vi "标准状态机.vi"(7 "Stop":bool, 8 "error in (no error)":errorcluster caption="错误输入（无错误）", 11 "Start":bool) -> (0 "error out":errorcluster caption="错误输出", 3 "Status":T1={"State"=enum."Idle", "Motor"={"#1"=FALSE, "#2"=FALSE, "#3"=FALSE}, "Timer"=30.0})   [LabVIEW 2013]
uses:
  Control/Data.ctl
  Control/State.ctl
  Control/Motor.ctl
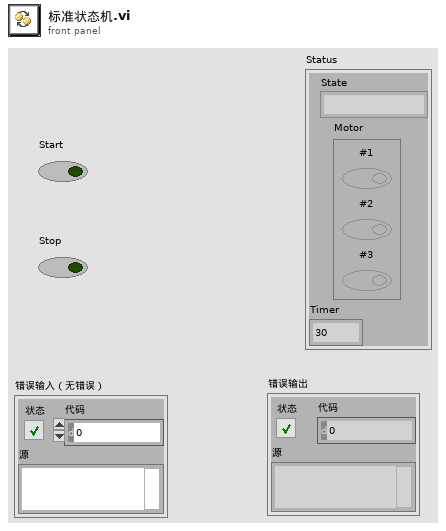
[diagram p1: front panel]
types:
  T1 = typedef "Data.ctl" = cluster{"State":T2, "Motor":T3, "Timer":dbl}
  T2 = typedef "State.ctl" = enum16{"Idle", "#1 Run", "#2 Run", "#3 Run", "#3 Stop", "#2 Stop", "#1 Stop"}
  T3 = typedef "Motor.ctl" = cluster{"#1":bool, "#2":bool, "#3":bool}
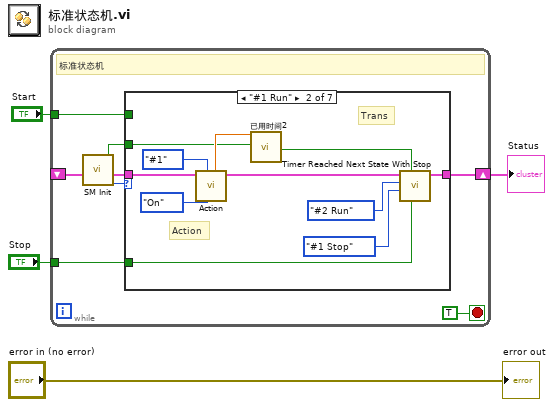
[diagram p0: block diagram]
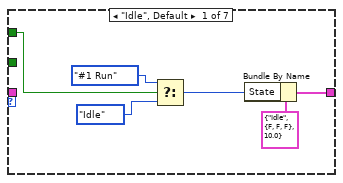
[diagram p2: hidden frame]
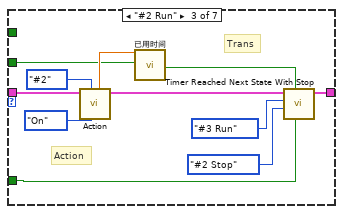
[diagram p3: hidden frame]
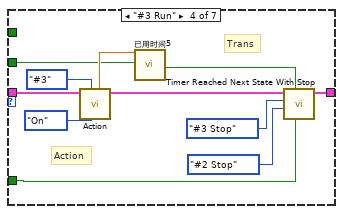
[diagram p4: hidden frame]
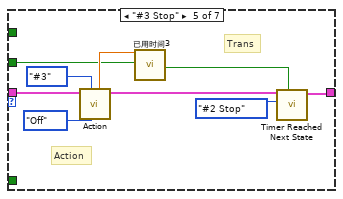
[diagram p5: hidden frame]
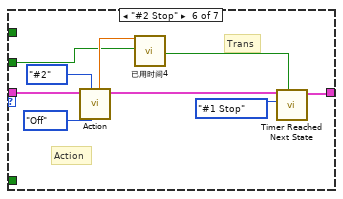
[diagram p6: hidden frame]
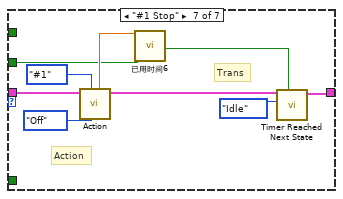
[diagram p7: hidden frame]
diagram:
  n1 = while {
    shift-right: [w11] -> w2
    shift-left: _ -> [w8]
    tunnel: "Start" -> [w12]
    tunnel: "Stop" -> [w9]
    stop <- TRUE stop-if-true
    # "标准状态机"
    n2 = call "SM Init.vi"("Status In"=w8) -> ("State"=w6:T2, "Status Out"=w7:T1, "State Changed"=w5:bool)  [unwired: 8 in]
    n3 = case shown="\"#1 Run\"" w6 {
      tunnel: w7 -> [_ w26 w37 w46 w60 w69 w78]
      tunnel: w12 -> [w15 _ _ _ _ _ _]
      tunnel: [w13 w27 w38 w47 w54 w63 w72] -> w11
      tunnel: w9 -> [_ w20 w31 w49 _ _ _]
      tunnel: w5 -> [_ w19 w30 w41 w52 w61 w70]
      frame "Idle", Default {
        n4 = Select(t=State."#1 Run" ("State"), s=w15, f=State."Idle" ("State")) -> (s? t:f=w14:T2)
        n5 = Bundle By Name(cluster=T1 {"State"=enum."Idle", "Motor"={"#1"=FALSE, "#2"=FALSE, "#3"=FALSE}, "Timer"=10.0} ("Status"), "State"=w14) -> (w13:T1)
      }
      frame "#1 Run" {
        # "Trans"
        # "Action"
        n6 = call "Action.vi"("On/Off"=enum16{"Off", "On"}."On", "Motor"=enum16{"#1", "#2", "#3"}."#1", "Data In"=w26) -> ("Data Out"=w25:T1, "Timer"=w24:dbl)  [unwired: 6 in, 1 out]
        n7 = call "已用时间2"("Time Target (s)"=w24, "Reset"=w19) -> ("Time has Elapsed"=w21:bool)  [unwired: 10 in, 7 out]
        n8 = call "Timer Reached Next State With Stop.vi"("Stop"=w20, "Time has Elapsed"=w21, "Stop State"=State."#1 Stop", "Next State"=State."#2 Run" ("State"), "Status Out输入"=w25) -> ("Status Out输出"=w27:T1)  [unwired: 6 in]
      }
      frame "#2 Run" {
        # "Trans"
        # "Action"
        n9 = call "Action.vi"("On/Off"=enum16{"Off", "On"}."On", "Motor"=enum16{"#1", "#2", "#3"}."#2", "Data In"=w37) -> ("Data Out"=w36:T1, "Timer"=w35:dbl)  [unwired: 6 in, 1 out]
        n10 = call "已用时间"("Time Target (s)"=w35, "Reset"=w30) -> ("Time has Elapsed"=w32:bool)  [unwired: 10 in, 7 out]
        n11 = call "Timer Reached Next State With Stop.vi"("Stop"=w31, "Time has Elapsed"=w32, "Stop State"=State."#2 Stop", "Next State"=State."#3 Run" ("State"), "Status Out输入"=w36) -> ("Status Out输出"=w38:T1)  [unwired: 6 in]
      }
      frame "#3 Run" {
        # "Trans"
        # "Action"
        n12 = call "Action.vi"("On/Off"=enum16{"Off", "On"}."On", "Motor"=enum16{"#1", "#2", "#3"}."#3", "Data In"=w46) -> ("Data Out"=w45:T1, "Timer"=w44:dbl)  [unwired: 6 in, 1 out]
        n13 = call "已用时间5"("Time Target (s)"=w44, "Reset"=w41) -> ("Time has Elapsed"=w48:bool)  [unwired: 10 in, 7 out]
        n14 = call "Timer Reached Next State With Stop.vi"("Stop"=w49, "Time has Elapsed"=w48, "Stop State"=State."#2 Stop", "Next State"=State."#3 Stop" ("State"), "Status Out输入"=w45) -> ("Status Out输出"=w47:T1)  [unwired: 6 in]
      }
      frame "#3 Stop" {
        # "Trans"
        # "Action"
        n15 = call "Action.vi"("On/Off"=enum16{"Off", "On"}."Off", "Motor"=enum16{"#1", "#2", "#3"}."#3", "Data In"=w60) -> ("Data Out"=w55:T1, "Timer"=w59:dbl)  [unwired: 6 in, 1 out]
        n16 = call "已用时间3"("Time Target (s)"=w59, "Reset"=w52) -> ("Time has Elapsed"=w56:bool)  [unwired: 10 in, 7 out]
        n17 = call "Timer Reached Next State.vi"("Time has Elapsed"=w56, "Next State"=State."#2 Stop", "Status Out输入"=w55) -> ("Status Out输出"=w54:T1)  [unwired: 8 in]
      }
      frame "#2 Stop" {
        # "Trans"
        # "Action"
        n18 = call "Action.vi"("On/Off"=enum16{"Off", "On"}."Off", "Motor"=enum16{"#1", "#2", "#3"}."#2", "Data In"=w69) -> ("Data Out"=w64:T1, "Timer"=w68:dbl)  [unwired: 6 in, 1 out]
        n19 = call "已用时间4"("Time Target (s)"=w68, "Reset"=w61) -> ("Time has Elapsed"=w65:bool)  [unwired: 10 in, 7 out]
        n20 = call "Timer Reached Next State.vi"("Time has Elapsed"=w65, "Next State"=State."#1 Stop", "Status Out输入"=w64) -> ("Status Out输出"=w63:T1)  [unwired: 8 in]
      }
      frame "#1 Stop" {
        # "Trans"
        # "Action"
        n21 = call "Action.vi"("On/Off"=enum16{"Off", "On"}."Off", "Motor"=enum16{"#1", "#2", "#3"}."#1", "Data In"=w78) -> ("Data Out"=w73:T1, "Timer"=w77:dbl)  [unwired: 6 in, 1 out]
        n22 = call "已用时间6"("Time Target (s)"=w77, "Reset"=w70) -> ("Time has Elapsed"=w74:bool)  [unwired: 10 in, 7 out]
        n23 = call "Timer Reached Next State.vi"("Time has Elapsed"=w74, "Next State"=State."Idle", "Status Out输入"=w73) -> ("Status Out输出"=w72:T1)  [unwired: 8 in]
      }
    }
  }
  "Status" <- w2
  "error out" <- "error in (no error)"
